vi "Page_Source_Can_Add_To_Bottom.vi"(8 "error in (no error)":errorcluster, 11 "AB_Source_PackedItem in":refnum<class "AB_Source_PackedItem.lvclass">) -> (0 "error out":errorcluster, 1 "message":string, 2 "canAddToBottom":bool, 3 "AB_Source_PackedItem out":refnum<class "AB_Source_PackedItem.lvclass">)   [LabVIEW 2020, in "AB_Source_PackedItem.lvclass"]
uses:
  <vilib>/AppBuilder/AB_Classes/Source/PackedItem/AB_Source_PackedItem.lvclass
  <resource>/Framework/Providers/Common/provcom_StringGlobals.vi
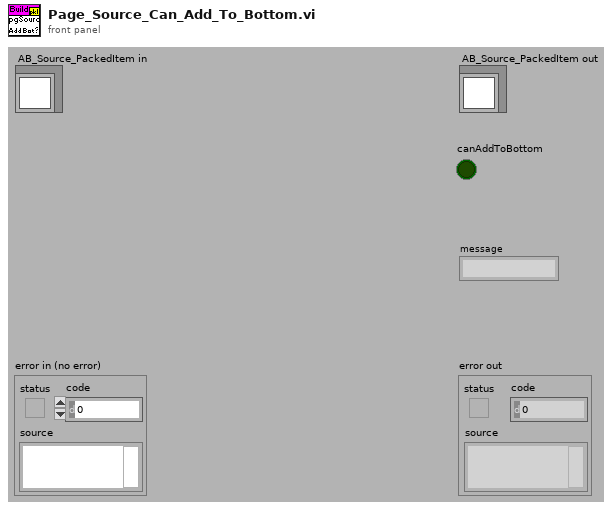
[diagram p1: front panel]
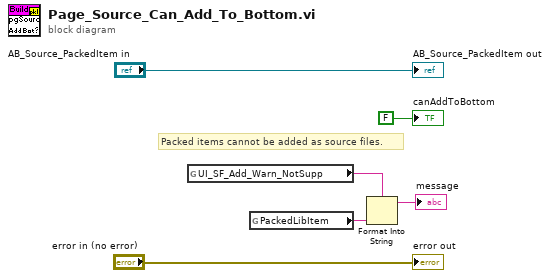
[diagram p0: block diagram]
diagram:
  # "Packed items cannot be added as source files."
  n1 = global read "provcom_StringGlobals.vi" "UI_SF_Add_Warn_NotSupp"() -> (w3:string)
  n2 = global read "provcom_StringGlobals.vi" "PackedLibItem"() -> (w1:string)
  n3 = Format Into String(format string=w3, w1) -> (resulting string=→"message":string)  [unwired: 2 in, 1 out]
  "error out" <- "error in (no error)"
  "AB_Source_PackedItem out" <- "AB_Source_PackedItem in"
  "canAddToBottom" <- FALSE ("canAddToBottom")
